vi "XIPIN_Divider_Generator_4_0.vi"   [LabVIEW 2017]
doc: "This core provides division using one of two algorithms. The Radix-2 algorithm provides a fabric solution suitable for smaller operand division, and High Radix algorithm provides a solution based upon XtremeDSP slices and so is well suited to larger operands (that is above about 16 bits wide).\n------------------------------------\n<b>Need License</b> : No\n<b>Interface</b> : AXI4-Stream"
uses:
  <vilib>/rvi/XilinxIP/XIPIN_XNode/niFpgaXIPIN.xnode
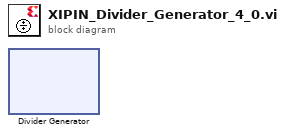
[diagram p0: block diagram]
diagram:
  n1 = xnode ("Divider Generator")() -> ()
